vi "63_Vision_RC Servo_c2.vi"() -> ()   [LabVIEW 2018]
uses:
  <userlib>/KNR OS 4.0 LabVIEW Toolkit/Type Definition/Resource.ctl
  <userlib>/KNR OS 4.0 LabVIEW Toolkit/Type Definition/RC Servo Port.ctl
panel:
  out "RC Pulse Width (uS)":u16[](array[numeric])
  out "Image Out":T1(plugin-control)
  in  "stop":bool
  # "找不到目標servo回中間"
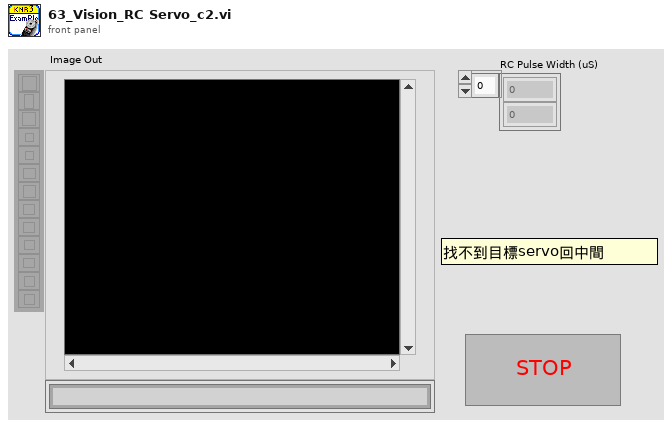
[diagram p1: front panel]
types:
  T1 = typedef "IMAQ Image.ctl" = refnum<image>
  T2 = typedef "RC Servo Port.ctl" = u16
  T3 = typedef "Resource.ctl" = enum16{"KNRm_DDRC", "KNRm_DDDD", "KNRm_DDDR", "KNRm_DDDC", "KNR", "KNRm_neww"}
  T4 = typedef "KNR3 Reference.ctl" = cluster{"FPGA Session":refnum<class "FPGA Interface Base.lvclass">, "Resource":T3}
  T5 = cluster{"Left":dbl, "Top":dbl, "Right":dbl, "Bottom":dbl}
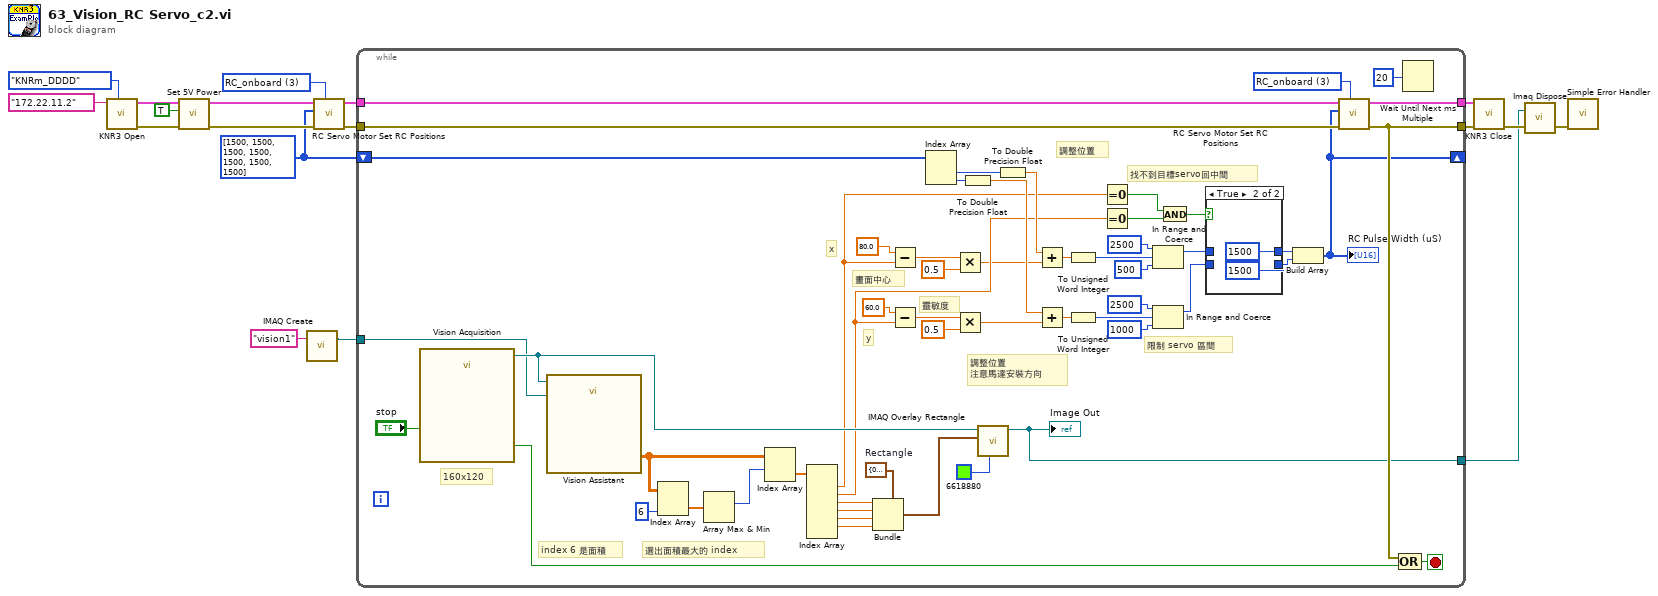
[diagram p0: block diagram]
diagram:
  w4 = u16[] [1500, 1500, 1500, 1500, 1500, 1500, 1500] ("RC Pulse Width (1500 uS)")
  w7 = T2 3 items=["RC_onboard"=3, "RC_box"=9] ("Port (RC_onboard)")
  n1 = call <userlib>:"KNR3 Open.vi"("Resource"=Resource."KNRm_DDDD", "IP"="172.22.11.2") -> ("error out"=w15:errorcluster, "KNR out"=w17:T4)  [unwired: 8 in]
  n2 = call <userlib>:"Set 5V Power.vi"("error in (no error)"=w15, "5V Power(T)"=TRUE ("5V Power"), "KNR in"=w17) -> ("error out"=w14:errorcluster, "KNR out"=w16:T4)  [unwired: 7 in]
  n3 = call "IMAQ Create"("Image Name"="vision1") -> ("New Image"=w5:T1)  [unwired: 4 in, 1 out]
  n4 = call <userlib>:"RC Servo Motor Set RC Positions.vi"("Port (RC_onboard)"=w7, "RC Pulse Width (1500 uS)"=w4, "KNR in"=w16) -> ("KNR out"=w8:T4)  [unwired: 7 in, 1 out]
  n5 = while {
    tunnel: w8 -> [w72]
    tunnel: [w71] -> w10
    tunnel: w14 -> [w70]
    tunnel: [w68] -> w9
    tunnel: w5 -> [w52]
    shift-right: [w36] -> _
    shift-left: w4 -> [w39]
    tunnel: [w18] -> w1
    stop <- w69 stop-if-true
    w64 = T5 {"Left"=0.0, "Top"=0.0, "Right"=0.0, "Bottom"=0.0}  # Rectangle
    w66 = T2 3 items=["RC_onboard"=3, "RC_box"=9] ("RC Motor")
    # "調整位置\n注意馬達安裝方向"
    # "index 6 是面積"
    # "調整位置"
    # "限制 servo 區間"
    # "靈敏度"
    # "畫面中心"
    # "找不到目標servo回中間"
    # "y"
    # "x"
    # "160x120"
    # "選出面積最大的 index"
    n6 = call "Vision Acquisition"("Stop (F)"="stop") -> ("Image Out"=w57:T1, "Stopped"=w50:bool)  [unwired: 24 in, 1 out]
    n7 = call "Vision Assistant"("Image In"=w57, "Image Dst"=w52) -> ("Particle Measurements (Pixels) (Particle Analysis 1)"=w56:dbl[][])  [unwired: 22 in, 3 out]
    n8 = Index Array "Index Array"(array=w56, index (col)=6 ("disabled index (col)")) -> (element=w55:dbl[])  [unwired: 1 in]
    n9 = Array Max & Min(array=w55) -> (max index (indices)=w54:i32)  [unwired: 3 out]
    n10 = Index Array "Index Array"(array=w56, index (row)=w54) -> (element=w65:dbl[])  [unwired: 1 in]
    n11 = Index Array "Index Array"(array=w65) -> (element #1=w29:dbl, element #2=w28:dbl, element #3=w63:dbl, element #4=w62:dbl, element #5=w61:dbl, element #6=w60:dbl)  [unwired: 7 in, 1 out]
    n12 = Bundle "Bundle"(cluster=w64, "Left"=w63, "Top"=w62, "Right"=w61, "Bottom"=w60) -> (w59:T5)
    n13 = Subtract(x=80.0 ("y"), y=w29) -> (x-y=w46:dbl)
    n14 = Subtract(x=60.0 ("y"), y=w28) -> (x-y=w47:dbl)
    n15 = Index Array "Index Array"(array=w39) -> (element #1=w38:u16, element #2=w37:u16)  [unwired: 2 in]
    n16 = Multiply(x=w46, y=0.5) -> (x*y=w27:dbl)
    n17 = Multiply(x=w47, y=0.5) -> (x*y=w26:dbl)
    n18 = To Double Precision Float(number=w37) -> (double precision float=w30:dbl)
    n19 = call "IMAQ Overlay Rectangle"("Color"=u32 6618880, "Rectangle"=w59, "Image"=w57) -> ("Image Out"=w18:T1)  [unwired: 7 in, 1 out]
    "Image Out" <- w18
    n20 = To Double Precision Float(number=w38) -> (double precision float=w31:dbl)
    n21 = Add(x=w31, y=w27) -> (x+y=w48:dbl)
    n22 = Add(x=w30, y=w26) -> (x+y=w49:dbl)
    n23 = To Unsigned Word Integer(number=w48) -> (unsigned 16bit integer=w33:u16)
    n24 = To Unsigned Word Integer(number=w49) -> (unsigned 16bit integer=w32:u16)
    n25 = Equal To 0?(x=w29) -> (x = 0?=w23:bool)
    n26 = Equal To 0?(x=w28) -> (x = 0?=w24:bool)
    n27 = In Range and Coerce(upper limit=u16 2500, x=w33, lower limit=u16 500) -> (coerced(x)=w22:u16)  [unwired: 1 out]
    n28 = In Range and Coerce(upper limit=u16 2500, x=w32, lower limit=u16 1000) -> (coerced(x)=w21:u16)  [unwired: 1 out]
    n29 = And(x=w23, y=w24) -> (x .and. y?=w25:bool)
    n30 = case shown="True" w25 {
      tunnel: w22 -> [w74 _]
      tunnel: w21 -> [w73 _]
      tunnel: [w74 u16 1500] -> w20
      tunnel: [w73 u16 1500] -> w19
      frame False {
      }
      frame True {
      }
    }
    n31 = Build Array(w20, w19) -> (w36:u16[])
    "RC Pulse Width (uS)" <- w36
    n32 = call <userlib>:"RC Servo Motor Set RC Positions.vi"("Port (RC_onboard)"=w66, "error in (no error)"=w70, "RC Pulse Width (1500 uS)"=w36, "KNR in"=w72) -> ("error out"=w68:errorcluster, "KNR out"=w71:T4)  [unwired: 6 in]
    n33 = Compound Arithmetic op=OR(w68, w50) -> (w69:bool)
    n34 = Wait Until Next ms Multiple(millisecond multiple=u32 20) -> ()  [unwired: 1 out]
  }
  n35 = call <userlib>:"KNR3 Close.vi"("error in (no error)"=w9, "KNR in"=w10) -> ("error out"=w3:errorcluster)  [unwired: 9 in]
  n36 = call "Imaq Dispose"("Image"=w1, "error in (no error)"=w3) -> ("error out"=w2:errorcluster)  [unwired: 4 in]
  n37 = call <vilib>:"Simple Error Handler.vi"("error in (no error)"=w2) -> ()  [unwired: 4 in, 5 out]
